vi "Load Config.vi"(8 "error in (no error)":errorcluster, 11 "VolatusConfig in":refnum<class "VolatusConfig.lvclass">) -> (0 "error out":errorcluster, 3 "VolatusConfig out":refnum<class "VolatusConfig.lvclass">, 5 "Config Path":path)   [LabVIEW 2023, in "VolatusConfig.lvlib" / "VolatusConfig.lvclass"]
uses:
  VolatusConfig.lvclass
  lv-web-crypto/lv-crypto/Crypto/Hashes/SHA-256/SHA-256.lvclass
  VolatusConfig.lvclass/VolatusConfig.ctl
  lv-cdm/CDM-Config/Config Storage/Config Storage.lvclass
  lv-web-crypto/lv-crypto/Crypto/Crypto.lvlib
  lv-cdm/CDM-Config/Config Manager/Config Manager.lvclass
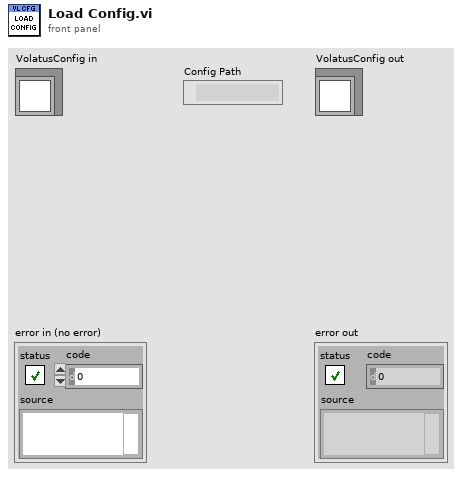
[diagram p1: front panel]
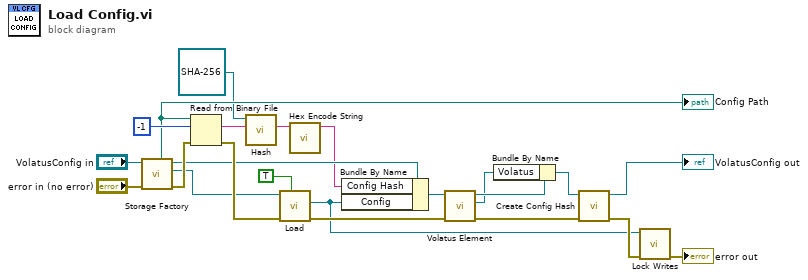
[diagram p0: block diagram]
diagram:
  n1 = call "Storage Factory.vi"("error in (no error)"="error in (no error)", "VolatusConfig in"="VolatusConfig in") -> ("error out"=w22:errorcluster, "Storage"=w17:refnum<class "Config Storage.lvclass">, "VolatusConfig out"=w18:refnum<class "VolatusConfig.lvclass">, "Config Path"=w15:path)  [unwired: 6 in]
  "Config Path" <- w15
  n2 = Read from Binary File(8:w22, 10:-1 ("count (1)"), 11:w15) -> (0:w21:errorcluster, 2:w8:string)  [unwired: 3 in, 2 out]
  n3 = call-dynamic "Hash.vi"("Message"=w8, "SHA-256 in"=refnum<class "SHA-256.lvclass"> refnum ("Crypto.lvlib:SHA-256.lvclass")) -> ("Hash"=w6:string)  [unwired: 7 in, 2 out]
  n4 = call "Load.vi"("Mutable (F)"=TRUE, "error in (no error)"=w21, "Config Storage in"=w17) -> ("error out"=w23:errorcluster, "Config"=w1:refnum<class "Config Manager.lvclass">)  [unwired: 6 in, 1 out]
  n5 = call "Hex Encode String.vi"("String"=w6) -> ("Hex Encoded String"=w5:string)  [unwired: 10 in]
  n6 = Bundle By Name(cluster=w18, "Config Hash"=w5, "Config"=w1) -> (w13:refnum<class "VolatusConfig.lvclass">)
  n7 = call "Volatus Element.vi"("error in (no error)"=w23, "VolatusConfig in"=w13) -> ("error out"=w4:errorcluster, "Volatus Element"=w9:refnum<class "Config Element.lvclass">, "VolatusConfig out"=w11:refnum<class "VolatusConfig.lvclass">)  [unwired: 7 in]
  n8 = Bundle By Name(cluster=w11, "Volatus"=w9) -> (w10:refnum<class "VolatusConfig.lvclass">)
  n9 = call "Create Config Hash.vi"("error in (no error)"=w4, "VolatusConfig in"=w10) -> ("error out"=w14:errorcluster, "VolatusConfig out"=→"VolatusConfig out":refnum<class "VolatusConfig.lvclass">)  [unwired: 8 in]
  n10 = call "Lock Writes.vi"("error in (no error)"=w14, "Config Manager in"=w1) -> ("error out"=→"error out":errorcluster)  [unwired: 8 in, 1 out]
